vi "VNA.vi"() -> ()   [LabVIEW 2022 SP3]
uses:
  <vilib>/Utility/file.llb/Write Delimited Spreadsheet (DBL).vi
  <instrlib>/VNA/Agilent ENA Series/Agilent ENA Series.lvlib
panel:
  in  "wait time (ms)":dbl
  in  "Smoothing State (F: Off)":bool
  in  "IF Bandwidth (100000.0)":dbl=100000.0 format="%^.1e"
  in  "Average Factor (16)":i32=16
  in  "Averaging State (F: Off)":bool
  in  "Continuous Sweep (T: Enable)":bool
  in  "Point Trigger (F: Disable)":bool
  in  "Trigger Source":u16(ring) items=["Internal", "External", "Manual", "BUS"]
  in  "Stop (MHz)":dbl format="%^.2e"
  in  "Start (Mhz)":dbl format="%^.2e"
  in  "Number of Measurement Points (201)":i32=201
  in  "Power Level (dBm)":dbl format="%^.2g"
  in  "file path (dialog if empty)":path
  in  "Measurement Parameters":u16(ring)=1 items=["S11", "S21", "S31", "S41", "S12", "S22", "S32", "S42", "S13", "S23", "S33", "S43", "S14", "S24", "S34", "S44", "A", "B", "C", "D", "R1", "R2", "R3", "R4"]
  out "Waveform Graph":dbl[](graph)
  in  "Safe Mode Maximum Power Level (30)":dbl=30.0
  in  "Safe Mode Minimum Power Level (-200)":dbl=-200.0
  in  "Tolerance Level (5)":dbl=5.0
  in  "Power Level Offset (0)":dbl
  in  "Port ( 1)":i32=1
  in  "Channel (1)":i32=1
  in  "Enable Safe Mode (T: Enabled)":bool=TRUE
  in  "Enable Receiver Leveling (T: Enabled)":bool=TRUE
  in  "Reset? (T: Yes)":bool=TRUE
  in  "ID Query? (T: Yes)":bool=TRUE
  in  "VISA resource name":refnum<visa-resource-name>
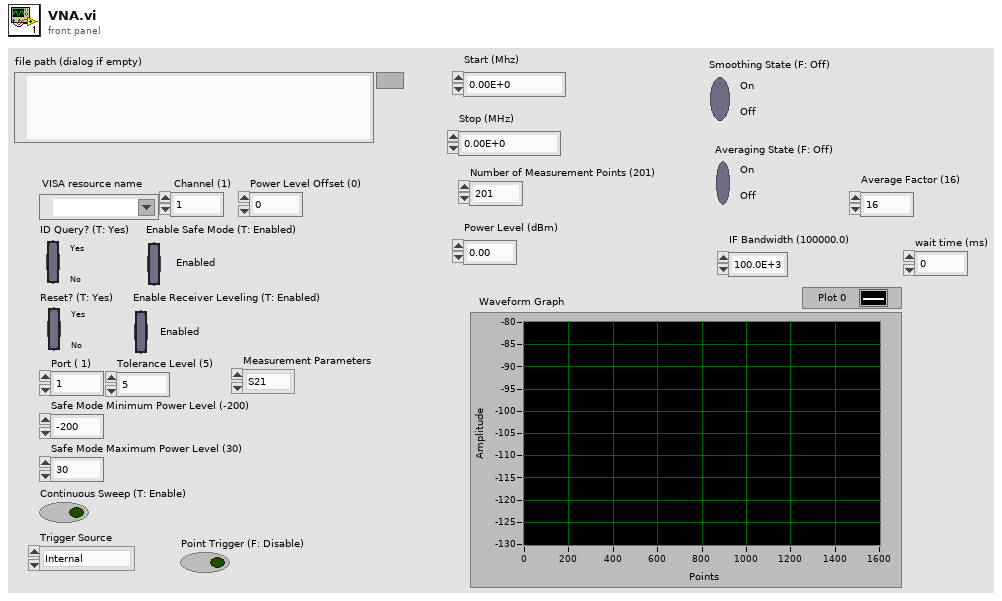
[diagram p1: front panel]
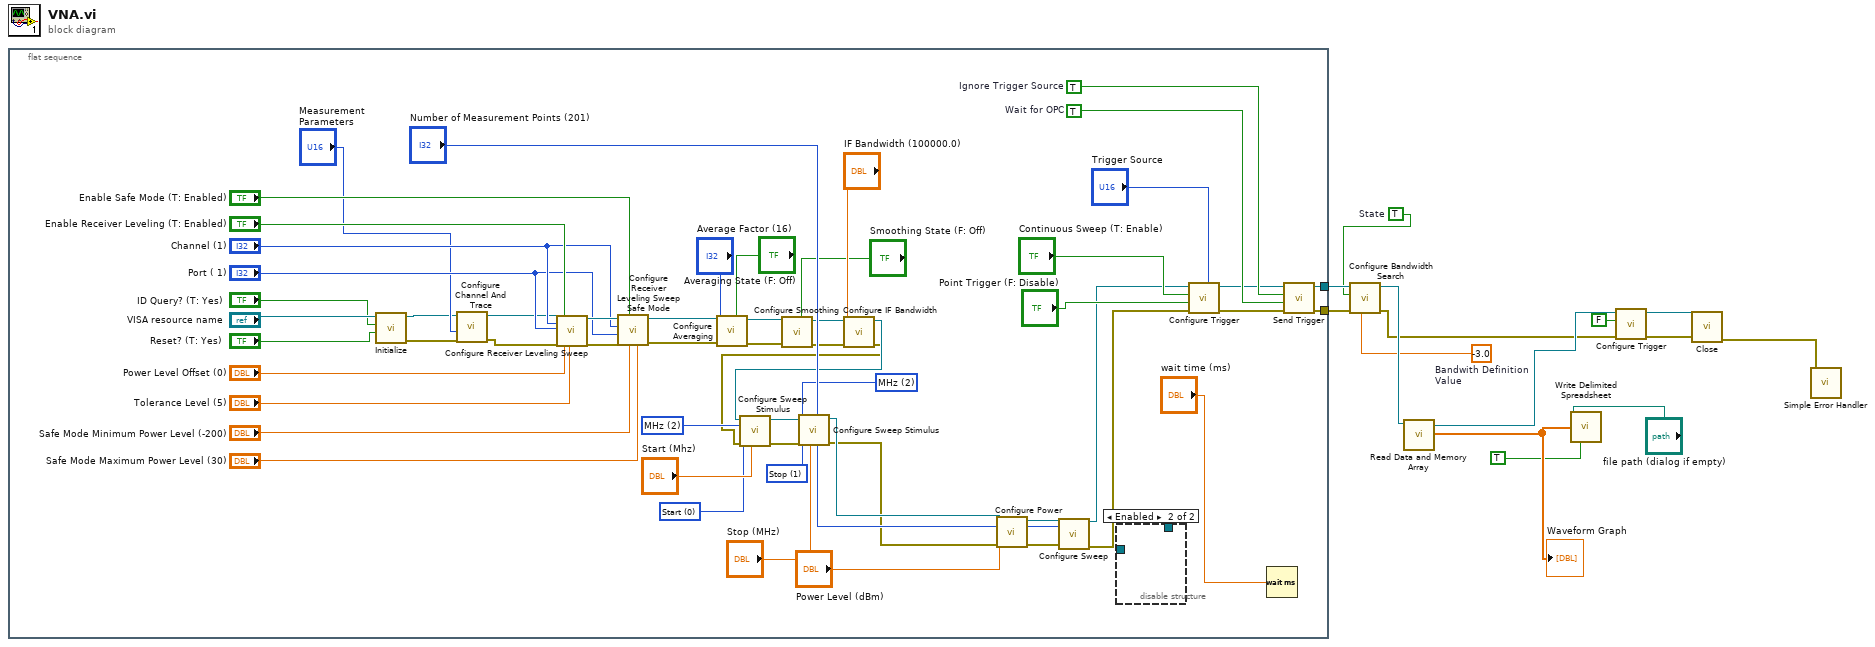
[diagram p0: block diagram]
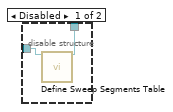
[diagram p2: hidden frame]
diagram:
  w4 = TRUE  # State
  w5 = -3.0  # Bandwith Definition Value
  n1 = flat-sequence {
    tunnel: [w68] -> w6
    tunnel: [w16] -> w3
    frame #0 {
      w43 = u16 2 items=["Hz", "kHz", "MHz", "GHz", "dBm", "s", "V"] ("Unit (0: Hz)")
      w44 = u16 2 items=["Hz", "kHz", "MHz", "GHz", "dBm", "s", "V"] ("Unit (0: Hz)")
      w45 = u16 1 items=["Start", "Stop", "Center", "Span"] ("Stimulus (0: Start)")
      w46 = u16 0 items=["Start", "Stop", "Center", "Span"] ("Stimulus (0: Start)")
      w69 = TRUE  # Wait for OPC
      w70 = TRUE  # Ignore Trigger Source
      n2 = call <instrlib>:"Initialize.vi"("Reset? (T: Yes)"="Reset? (T: Yes)", "ID Query? (T: Yes)"="ID Query? (T: Yes)", "VISA resource name"="VISA resource name") -> ("error out"=w28:errorcluster, "VISA resource name out"=w32:refnum<visa-resource-name>)  [unwired: 7 in]
      n3 = call <instrlib>:"Configure Channel And Trace.vi"("error in (no error)"=w28, "Measurement Parameters (0: S11)"="Measurement Parameters", "VISA resource name"=w32) -> ("error out"=w27:errorcluster, "VISA resource name out"=w31:refnum<visa-resource-name>)  [unwired: 7 in]
      n4 = call <instrlib>:"Configure Receiver Leveling Sweep.vi"("VISA resource name"=w31, "Channel (1)"="Channel (1)", "Port ( 1)"="Port ( 1)", "error in (no error)"=w27, "Enable Receiver Leveling (F: Disabled)"="Enable Receiver Leveling (T: Enabled)", "Power Level Offset (0)"="Power Level Offset (0)", "Tolerance Level (5)"="Tolerance Level (5)") -> ("VISA resource name out"=w63:refnum<visa-resource-name>, "error out"=w26:errorcluster)  [unwired: 11 in]
      n5 = call <instrlib>:"Configure Receiver Leveling Sweep Safe Mode.vi"("Safe Mode Maximum Power Level (30)"="Safe Mode Maximum Power Level (30)", "Safe Mode Minimum Power Level (-200)"="Safe Mode Minimum Power Level (-200)", "Enable Safe Mode (F: Disabled)"="Enable Safe Mode (T: Enabled)", "error in (no error)"=w26, "Port ( 1)"="Port ( 1)", "Channel (1)"="Channel (1)", "VISA resource name"=w63) -> ("error out"=w25:errorcluster, "VISA resource name out"=w30:refnum<visa-resource-name>)  [unwired: 3 in]
      n6 = call <instrlib>:"Configure Averaging.vi"("Averaging State (F: Off)"="Averaging State (F: Off)", "error in (no error)"=w25, "Factor (16)"="Average Factor (16)", "VISA resource name"=w30) -> ("error out"=w24:errorcluster, "VISA resource name out"=w39:refnum<visa-resource-name>)  [unwired: 6 in]
      n7 = call <instrlib>:"Configure Smoothing.vi"("Smoothing State (F: Off)"="Smoothing State (F: Off)", "error in (no error)"=w24, "VISA resource name"=w39) -> ("error out"=w23:errorcluster, "VISA resource name out"=w38:refnum<visa-resource-name>)  [unwired: 7 in]
      n8 = call <instrlib>:"Configure IF Bandwidth.vi"("error in (no error)"=w23, "IF Bandwidth (100000.0)"="IF Bandwidth (100000.0)", "VISA resource name"=w38) -> ("error out"=w22:errorcluster, "VISA resource name out"=w37:refnum<visa-resource-name>)  [unwired: 7 in]
      n9 = call <instrlib>:"Configure Sweep Stimulus.vi"("Parameter (0.0)"="Start (Mhz)", "error in (no error)"=w22, "Stimulus (0: Start)"=w46, "Unit (0: Hz)"=w44, "VISA resource name"=w37) -> ("error out"=w21:errorcluster, "VISA resource name out"=w50:refnum<visa-resource-name>)  [unwired: 5 in]
      n10 = call <instrlib>:"Configure Sweep Stimulus.vi"("Parameter (0.0)"="Stop (MHz)", "error in (no error)"=w21, "Stimulus (0: Start)"=w45, "Unit (0: Hz)"=w43, "VISA resource name"=w50) -> ("error out"=w20:errorcluster, "VISA resource name out"=w49:refnum<visa-resource-name>)  [unwired: 5 in]
      n11 = call <instrlib>:"Configure Power.vi"("VISA resource name"=w49, "Power Level (0.0)"="Power Level (dBm)", "error in (no error)"=w20) -> ("VISA resource name out"=w52:refnum<visa-resource-name>, "error out"=w19:errorcluster)  [unwired: 11 in]
      n12 = call <instrlib>:"Configure Sweep.vi"("VISA resource name"=w52, "Number of Measurement Points (201)"="Number of Measurement Points (201)", "error in (no error)"=w19) -> ("VISA resource name out"=w29:refnum<visa-resource-name>, "error out"=w18:errorcluster)  [unwired: 11 in]
      n13 = disable-structure shown="Enabled" {
        disable-tunnel: _ -> [w72 _]
        disable-tunnel: [w71 _] -> _
        frame Disabled {
          n14 = call <instrlib>:"Define Sweep Segments Table.vi"("VISA resource name"=w72) -> ("VISA resource name out"=w71:refnum<visa-resource-name>)  [unwired: 17 in, 1 out]
        }
        frame Enabled {
        }
      }
      n15 = call <instrlib>:"Configure Trigger.vi"("Trigger Source (0: Internal)"="Trigger Source", "error in (no error)"=w18, "Point Trigger (F: Disable)"="Point Trigger (F: Disable)", "Continuous Sweep (T: Enable)"="Continuous Sweep (T: Enable)", "VISA resource name"=w29) -> ("error out"=w17:errorcluster, "VISA resource name out"=w64:refnum<visa-resource-name>)  [unwired: 5 in]
      n16 = Wait (ms)(milliseconds to wait="wait time (ms)") -> ()  [unwired: 1 out]
      n17 = call <instrlib>:"Send Trigger.vi"("error in (no error)"=w17, "Wait for OPC (F: Do not Wait)"=w69, "Ignore Trigger Source (F: Do not Ignore)"=w70, "VISA resource name"=w64) -> ("error out"=w16:errorcluster, "VISA resource name out"=w68:refnum<visa-resource-name>)  [unwired: 6 in]
    }
  }
  n18 = call <instrlib>:"Configure Bandwidth Search.vi"("Bandwidth Definition Value (-3.0)"=w5, "error in (no error)"=w3, "Result Display State (F: Disable)"=w4, "VISA resource name"=w6) -> ("error out"=w2:errorcluster, "VISA resource name out"=w7:refnum<visa-resource-name>)  [unwired: 6 in]
  n19 = call <instrlib>:"Read Data and Memory Array.vi"("VISA resource name"=w7) -> ("Primary / Real"=w13:dbl[], "VISA resource name out"=w10:refnum<visa-resource-name>)  [unwired: 7 in, 2 out]
  "Waveform Graph" <- w13
  n20 = call-poly <vilib>:"Write Delimited Spreadsheet.vi"("file path (dialog if empty)"="file path (dialog if empty)", "1D data"=w13, "transpose? (no:F)"=TRUE) -> ()  [unwired: 11 in, 2 out]
  n21 = call <instrlib>:"Configure Trigger.vi"("error in (no error)"=w2, "Continuous Sweep (T: Enable)"=FALSE, "VISA resource name"=w10) -> ("error out"=w1:errorcluster, "VISA resource name out"=w9:refnum<visa-resource-name>)  [unwired: 7 in]
  n22 = call <instrlib>:"Close.vi"("error in (no error)"=w1, "VISA resource name"=w9) -> ("error out"=w14:errorcluster)  [unwired: 9 in]
  n23 = call <vilib>:"Simple Error Handler.vi"("error in (no error)"=w14) -> ()  [unwired: 4 in, 5 out]
